vi "DAQ setting.vi"(8 "error in (no error)":errorcluster, 11 "vi reference":refnum<vi>) -> (0 "error Out":errorcluster, 3 "Out reference":refnum<vi>)   [LabVIEW 2015]
uses:
  Control Button/Exit.ctl
  Control Button/Save.ctl
  <vilib>/addons/database/Connection.llb/DB Tools Open Connec (String).vi
  <vilib>/addons/database/_DB Variant To Data/Database Variant To Data.xnode
  <vilib>/addons/database/NI_Database_API.lvlib
panel:
  out "error out":errorcluster
  in  "read":bool
  out "subarray":string[](array[string])
  in  "Save":T1
  in  "Exit":T2
  in  "Tab Control":T3(tab)
  in  "DAQmx OutPut Setting":T4
  in  "DAQmx InPut Setting":T5
  in  "DAQmx Analog Input Setting":T6
  in  "DAQmx  Counter In":tag
  in  "DAQmx  Counter In":tag
  in  "DAQmx Counter Out":tag
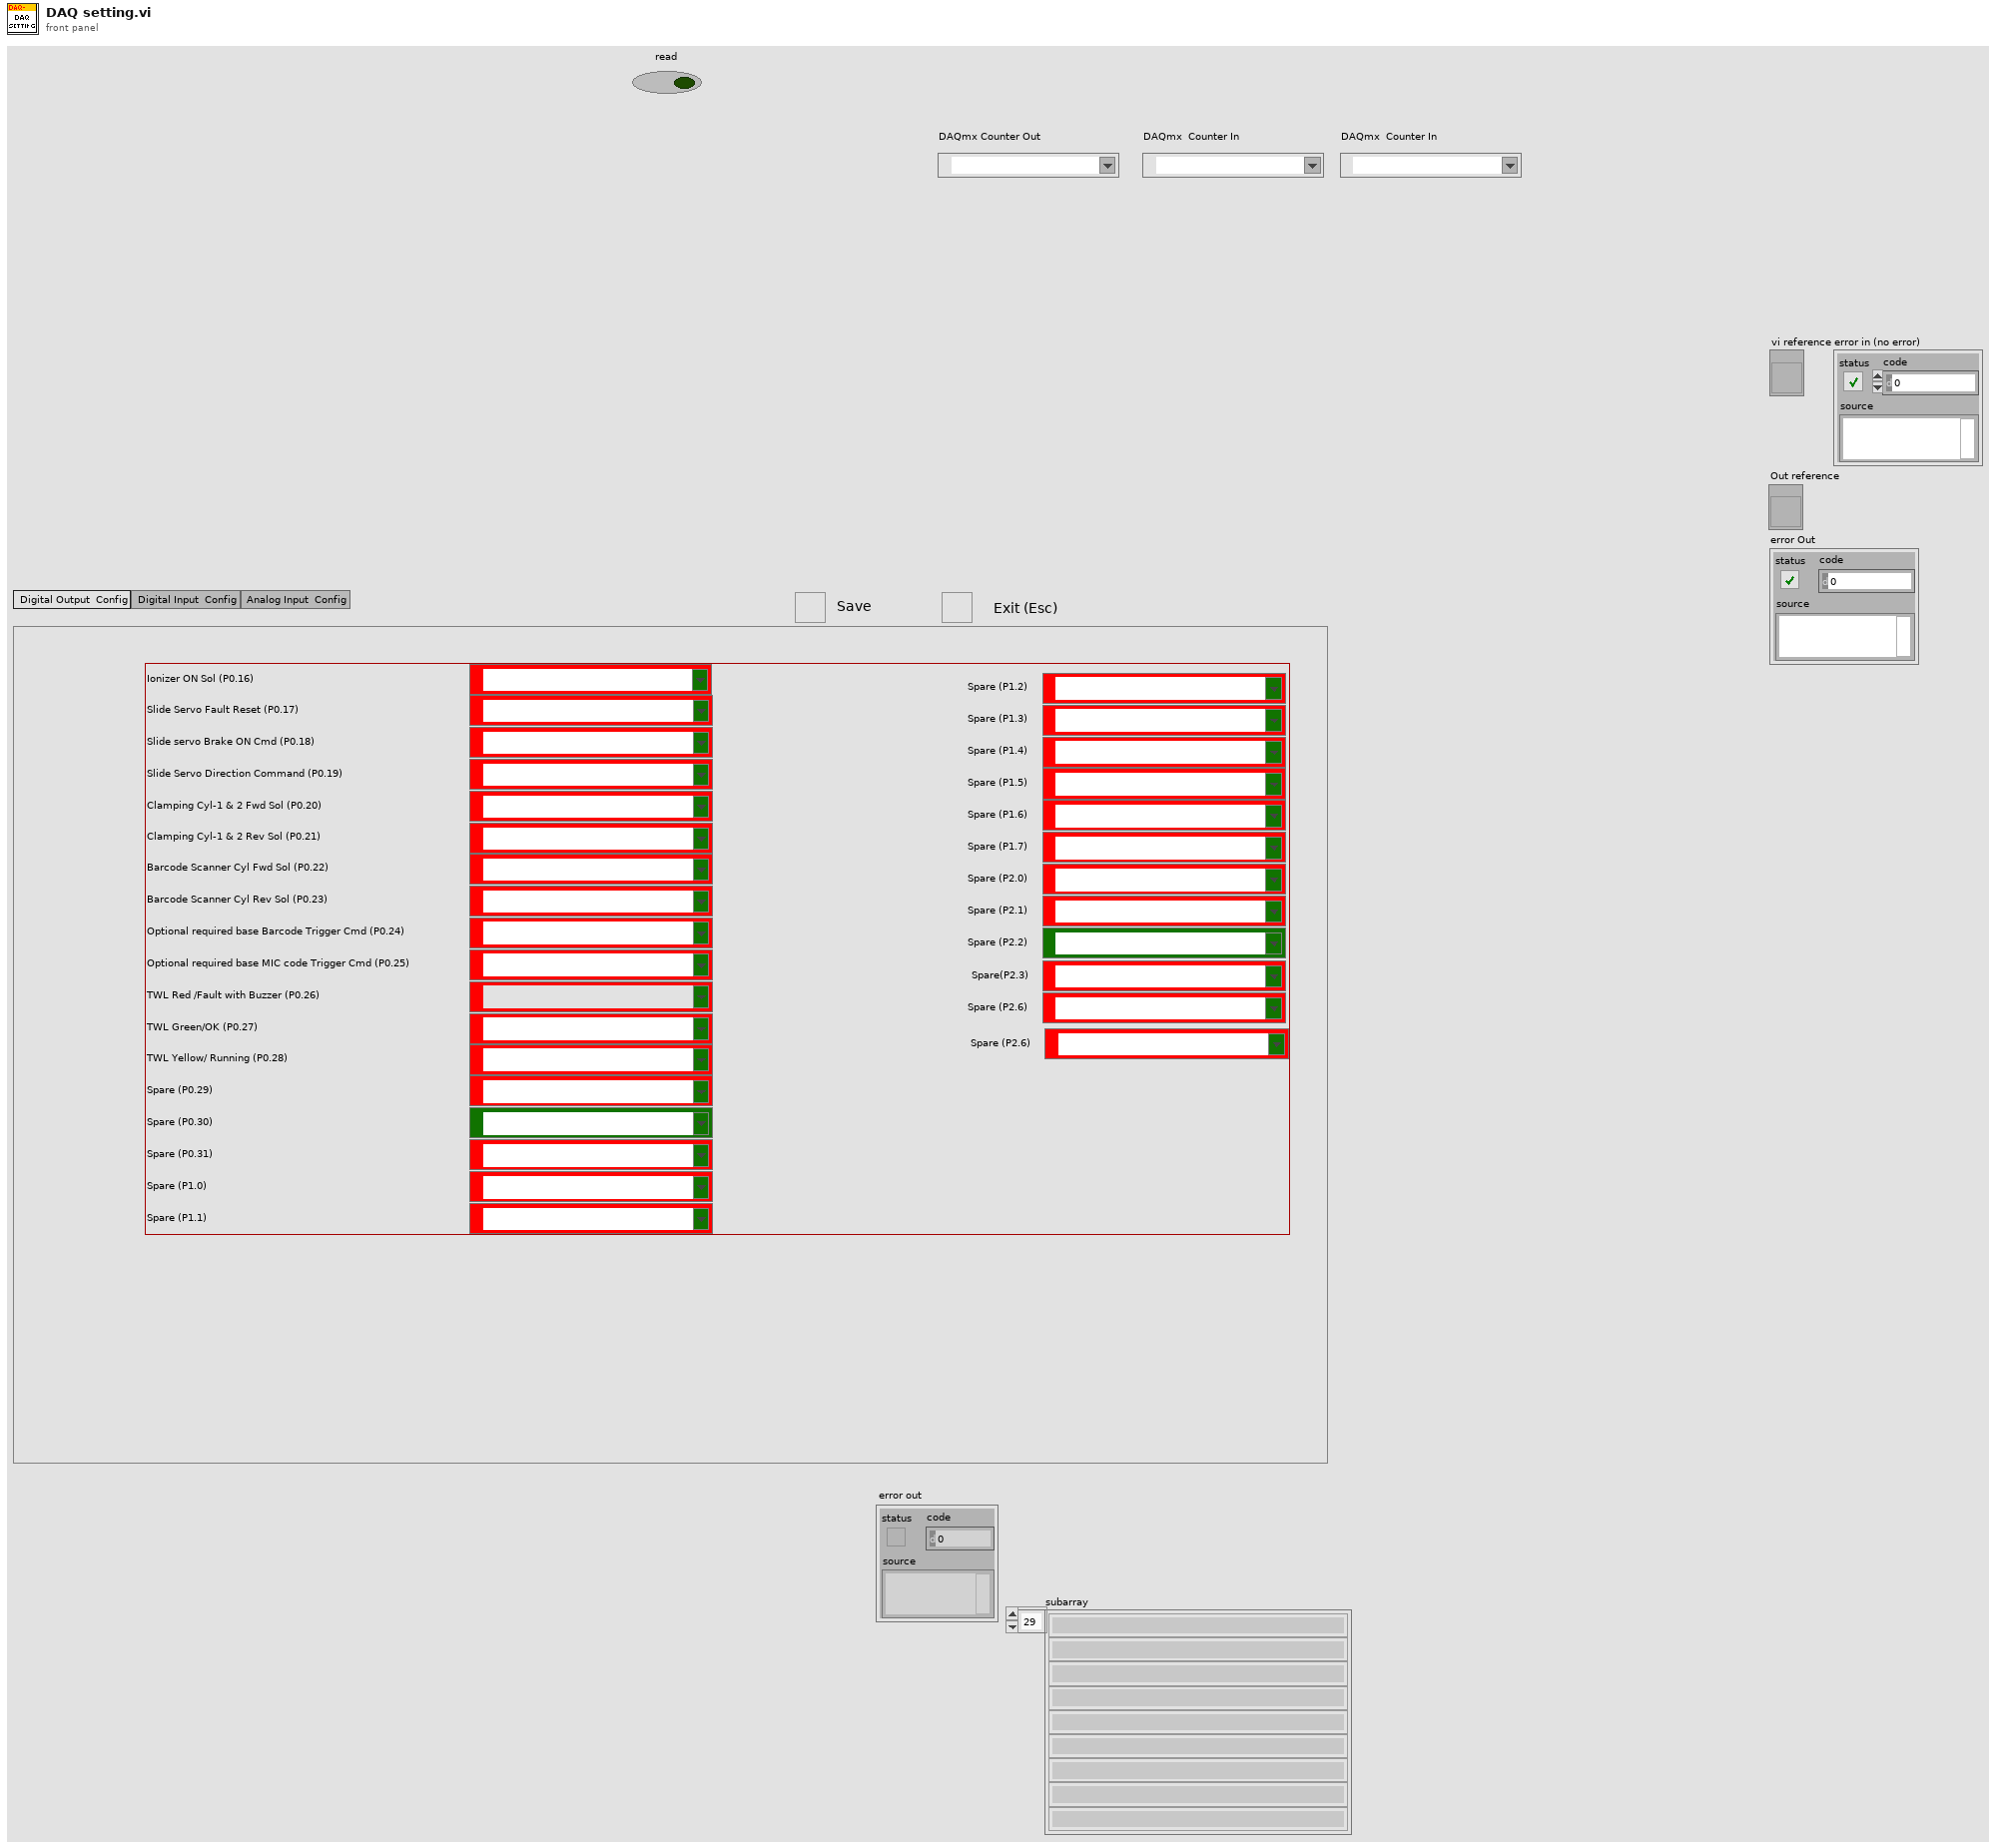
[diagram p1: front panel]
types:
  T1 = typedef "Save.ctl" = bool
  T2 = typedef "Exit.ctl" = bool
  T3 = enum32{"Digital Output  Config", "Digital Input  Config", "Analog Input  Config"}
  T4 = cluster{"DAQmx OutPut_00":tag, "DAQmx OutPut_01":tag, "DAQmx OutPut_02":tag, "DAQmx OutPut_03":tag, "DAQmx OutPut_04":tag, "DAQmx OutPut_05":tag, "DAQmx OutPut_06":tag, "DAQmx OutPut_07":tag, "DAQmx OutPut_08":tag, "DAQmx OutPut_09":tag, "DAQmx OutPut_10":tag, "DAQmx OutPut_11":tag, "DAQmx OutPut_12":tag, "DAQmx OutPut_13":tag, "DAQmx OutPut_14":tag, "DAQmx OutPut_15":tag, "DAQmx OutPut_16":tag, "DAQmx OutPut_17":tag, "DAQmx OutPut_18":tag, "DAQmx OutPut_19":tag, "DAQmx OutPut_20":tag, "DAQmx OutPut_21":tag, "DAQmx OutPut_22":tag, "DAQmx OutPut_23":tag, "DAQmx OutPut_12 2":tag, "DAQmx OutPut_13 2":tag, "DAQmx OutPut_14 2":tag, "DAQmx OutPut_15 2":tag, "DAQmx OutPut_16 2":tag, "String":string, "DAQmx OutPut_16 3":tag}
  T5 = cluster{"DAQmx InPut_00":tag, "DAQmx InPut_01":tag, "DAQmx InPut_02":tag, "DAQmx InPut_03":tag, "DAQmx InPut_04":tag, "DAQmx InPut_05":tag, "DAQmx InPut_06":tag, "DAQmx InPut_07":tag, "DAQmx InPut_08":tag, "DAQmx InPut_09":tag, "DAQmx InPut_10":tag, "DAQmx InPut_11":tag, "DAQmx InPut_12":tag, "DAQmx InPut_13":tag, "DAQmx InPut_14":tag, "DAQmx InPut_15":tag, "Key":string}
  T6 = cluster{"DAQmx Analog Input_00":tag, "DAQmx Analog Input_01":tag, "DAQmx Analog Input_02":tag, "DAQmx Analog Input_03":tag, "DAQmx Analog Input_04":tag, "DAQmx Analog Input_05":tag, "DAQmx Analog Input_06":tag, "DAQmx Analog Input_07":tag, "DAQmx Analog Input_08":tag, "DAQmx Analog Input_09":tag, "DAQmx Analog Input_10":tag, "DAQmx Analog Input_11":tag, "DAQmx Analog Input_12":tag, "DAQmx Analog Input_13":tag, "DAQmx Analog Input_14":tag, "DAQmx Analog Input_15":tag, "DAQmx Analog Input_16":tag, "DAQmx Analog Input_17":tag, "DAQmx Analog Input_18":tag, "DAQmx Analog Input_19":tag, "DAQmx Analog Input_20":tag, "DAQmx Analog Input_21":tag, "DAQmx Analog Input_22":tag, "DAQmx Analog Input_23":tag, "DAQmx Analog Input_24":tag, "DAQmx Analog Input_25":tag, "DAQmx Analog Input_26":tag, "DAQmx Analog Input_27":tag, "DAQmx Analog Input_28":tag, "DAQmx Analog Input_29":tag, "DAQmx Analog Input_30":tag, "DAQmx Analog Input_31":tag, "String 2":string}
  T7 = enum8{"Enabled", "Disabled", "Disabled and Grayed Out"}
  T8 = typedef "NI_Database_API.lvlib/Conn ObjectReference.ctl" = refnum<k1>
  T9 = cluster{"data[0]":string, "data[1]":string, "data[2]":string, "data[3]":string, "data[4]":string, "data[5]":string, "data[6]":string, "data[7]":string, "data[8]":string, "data[9]":string, "data[10]":string, "data[11]":string, "data[12]":string, "data[13]":string, "data[14]":string, "data[15]":string, "data[16]":string}
  T10 = cluster{"data[0]":string, "data[1]":string, "data[2]":string, "data[3]":string, "data[4]":string, "data[5]":string, "data[6]":string, "data[7]":string, "data[8]":string, "data[9]":string, "data[10]":string, "data[11]":string, "data[12]":string, "data[13]":string, "data[14]":string, "data[15]":string, "data[16]":string, "data[17]":string, "data[18]":string, "data[19]":string, "data[20]":string, "data[21]":string, "data[22]":string, "data[23]":string, "data[24]":string, "data[25]":string, "data[26]":string, "data[27]":string, "data[28]":string, "data[29]":string, "data[30]":string}
  T11 = cluster{"data[0]":string, "data[1]":string, "data[2]":string, "data[3]":string, "data[4]":string, "data[5]":string, "data[6]":string, "data[7]":string, "data[8]":string, "data[9]":string, "data[10]":string, "data[11]":string, "data[12]":string, "data[13]":string, "data[14]":string, "data[15]":string, "data[16]":string, "data[17]":string, "data[18]":string, "data[19]":string, "data[20]":string, "data[21]":string, "data[22]":string, "data[23]":string, "data[24]":string, "data[25]":string, "data[26]":string, "data[27]":string, "data[28]":string, "data[29]":string, "data[30]":string, "data[31]":string, "data[32]":string}
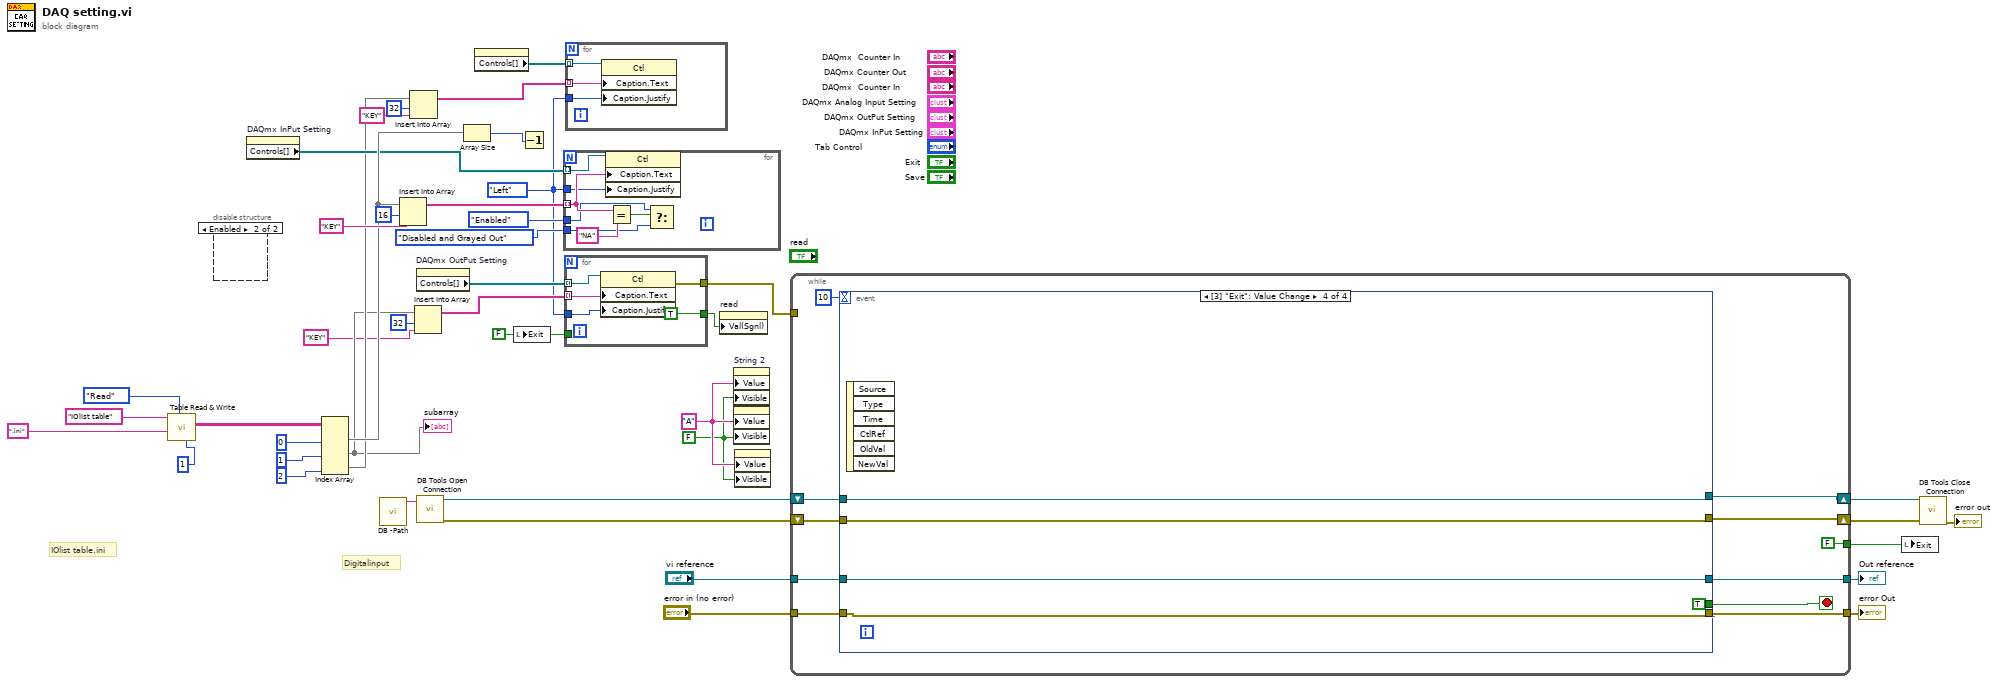
[diagram p0: block diagram]
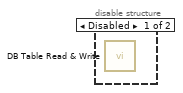
[diagram p2: hidden frame]
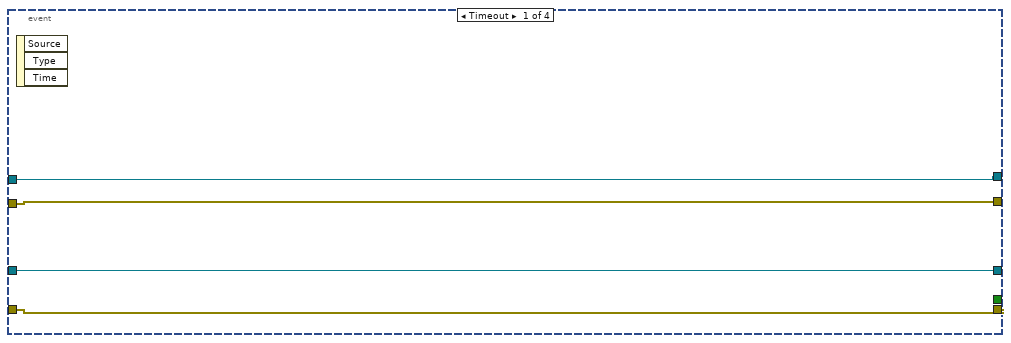
[diagram p3: hidden frame]
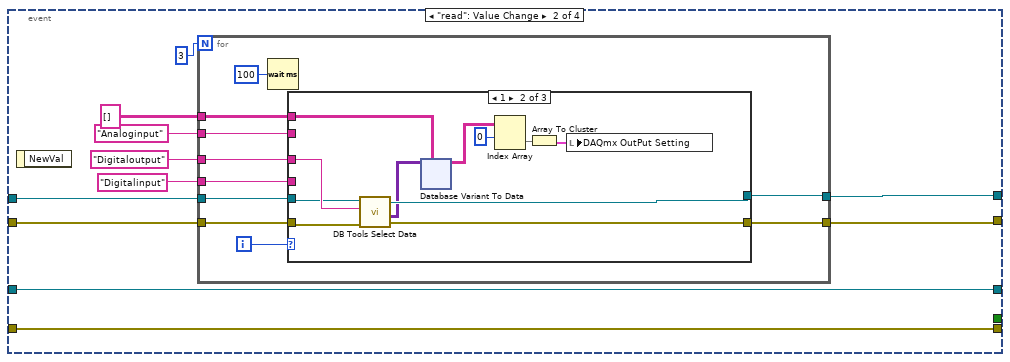
[diagram p4: hidden frame]
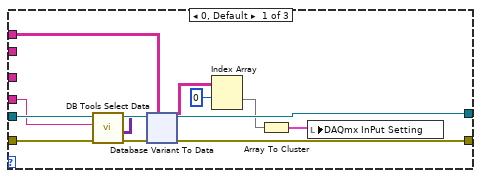
[diagram p5: hidden frame]
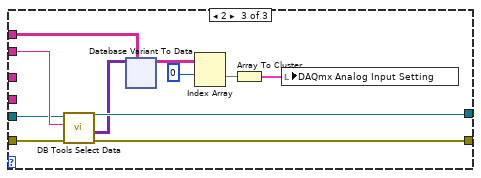
[diagram p6: hidden frame]
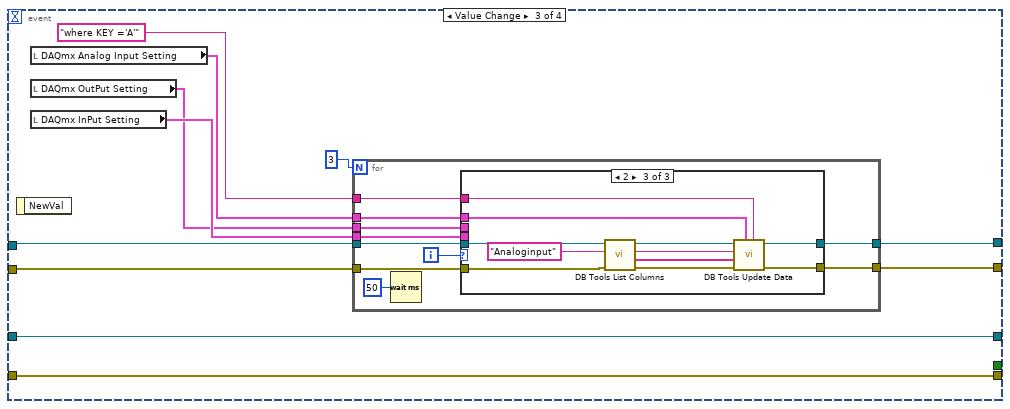
[diagram p7: hidden frame]
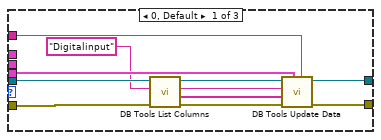
[diagram p8: hidden frame]
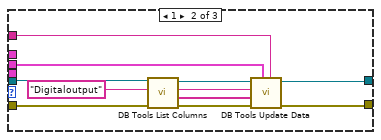
[diagram p9: hidden frame]
diagram:
  w1 = enum16{"Left", "Center", "Right"}."Left" ("Caption.Justification")
  w2 = FALSE ("Visible")
  w3 = "A" ("Value")
  w34 = T2 FALSE ("Exit")
  # "IOlist table.ini"
  # "Digitalinput"
  n1 = call "Table Read & Write.vi"("File Name"="IOlist table", "File type"=".ini", "Enum"=enum16{"Read", "Write"}."Read", "index"=1) -> ("Read Table"=w30:string[][])  [unwired: 5 in, 1 out]
  n2 = disable-structure shown="Enabled" {
    frame Disabled {
      n3 = call "DB Table Read & Write.vi"() -> ()  [unwired: 10 in, 2 out]
    }
    frame Enabled {
    }
  }
  n4 = property on="DAQmx InPut Setting" class="Clust (strict)"() -> ("Controls[]"=w13:refnum<vi>[])  [unwired: 2 in, 2 out]
  n5 = Index Array(array=w30, index (col) #1=0 ("disabled index (col)"), index (col) #2=1 ("index (col)"), index (col) #3=2 ("index (col)")) -> (element #1=w15:string[], element #2=w9:string[], element #3=w11:string[])  [unwired: 3 in]
  "subarray" <- w9
  n6 = call "DB -Path.vi"() -> ("String"=w27:string)  [unwired: 11 in]
  n7 = Insert Into Array(array=w15, index=16, new element="KEY" ("new element/subarray")) -> (w14:string[])
  n8 = Insert Into Array(array=w11, index=32, new element="KEY" ("new element/subarray")) -> (w4:string[])
  n9 = Insert Into Array(array=w9, index=32, new element="KEY" ("new element/subarray")) -> (w6:string[])
  n10 = property on="DAQmx OutPut Setting" class="Clust (strict)"() -> ("Controls[]"=w40:refnum<vi>[])  [unwired: 2 in, 2 out]
  n11 = call-poly <vilib>:"DB Tools Open Connection.vi"("connection information"=w27) -> ("error out"=w25:errorcluster, "connection reference"=w26:T8)  [unwired: 7 in]
  n12 = Array Size(array=w15) -> (size(s)=w18:i32)
  n13 = property on="DAQmx Analog Input Setting" class="Clust (strict)"() -> ("Controls[]"=w5:refnum<vi>[])  [unwired: 2 in, 2 out]
  n14 = local write "Exit"(w34) -> ()
  n15 = Decrement(x=w18) -> ()  [unwired: 1 out]
  n16 = for {
    tunnel: w13 -> [w50] mode=indexing
    tunnel: w14 -> [w48] mode=indexing
    tunnel: T7."Enabled" ("Disabled") -> [w47]
    tunnel: T7."Disabled and Grayed Out" ("Disabled") -> [w46]
    tunnel: w1 -> [w44]
    n17 = property class="Ctl"(reference=w50, "Caption.Text"=w48, "Caption.Justify"=w44) -> ()  [unwired: 1 in, 2 out]
    n18 = Equal?(x=w48, y="NA") -> (x = y?=w45:bool)
    n19 = Select(t=w47, s=w45, f=w46) -> ()  [unwired: 1 out]
  }
  n20 = for {
    tunnel: w40 -> [w55] mode=indexing
    tunnel: w6 -> [w54] mode=indexing
    tunnel: w34 -> [_]
    tunnel: [w53] -> w29
    tunnel: [TRUE] -> w28
    tunnel: w1 -> [w51]
    n21 = property class="Ctl"(reference=w55, "Caption.Text"=w54, "Caption.Justify"=w51) -> (error out=w53:errorcluster)  [unwired: 1 in, 1 out]
  }
  n22 = for {
    tunnel: w5 -> [w58] mode=indexing
    tunnel: w4 -> [w57] mode=indexing
    tunnel: w1 -> [w56]
    n23 = property class="Ctl"(reference=w58, "Caption.Text"=w57, "Caption.Justify"=w56) -> ()  [unwired: 1 in, 2 out]
  }
  n24 = property on="read" class="Bool (strict)"("Val(Sgnl)"=w28) -> ()  [unwired: 2 in, 2 out]
  n25 = property on="String 2" class="Str"("Value"=w3, "Visible"=w2) -> ()  [unwired: 2 in, 2 out]
  n26 = property on="Key" class="Str"("Value"=w3, "Visible"=w2) -> ()  [unwired: 2 in, 2 out]
  n27 = property on="String" class="Str"("Value"=w3, "Visible"=w2) -> ()  [unwired: 2 in, 2 out]
  n28 = while {
    tunnel: [FALSE] -> w39
    tunnel: "vi reference" -> [w66]
    tunnel: "error in (no error)" -> [w65]
    tunnel: [w64] -> w36
    tunnel: [w63] -> w35
    tunnel: w29 -> [_]
    shift-right: [w60] -> w24
    shift-left: w26 -> [w62]
    shift-right: [w59] -> w23
    shift-left: w25 -> [w61]
    stop <- w68 stop-if-true
    n29 = event shown="[3] \"Exit\": Value Change" {
      selector: _ -> [_ _ _ _]
      dyn-events: _ -> [_ _ _ _]
      timeout: 10 -> [_ _ _ _]
      tunnel: [_ _ _ TRUE] -> w68
      tunnel: w66 -> [w73 w84 w271 w315]
      tunnel: w65 -> [w72 w83 w270 w314]
      tunnel: [w73 w84 w271 w315] -> w64
      tunnel: [w72 w83 w270 w314] -> w63
      tunnel: w62 -> [w71 w77 w269 w313]
      tunnel: w61 -> [w70 w76 w268 w312]
      tunnel: [w71 w79 w266 w313] -> w60
      tunnel: [w70 w78 w265 w312] -> w59
      event Timeout {
        n30 = event-data() -> ()  [unwired: 1 in, 3 out]
      }
      event "read": Value Change {
        n31 = event-data() -> ()  [unwired: 1 in, 1 out]
        n32 = for {
          N: 3 -> [_]
          tunnel: "Digitalinput" ("table") -> [w92]
          tunnel: w77 -> [w91]
          tunnel: w76 -> [w90]
          tunnel: [w89] -> w79
          tunnel: [w88] -> w78
          tunnel: "Digitaloutput" ("table") -> [w87]
          tunnel: "Analoginput" ("table") -> [w86]
          tunnel: string[][] [] -> [w85]
          i -> [w94]
          n33 = Wait (ms)(milliseconds to wait=u32 100) -> ()  [unwired: 1 out]
          n34 = case shown="1" w94 {
            tunnel: w92 -> [w100 _ _]
            tunnel: w91 -> [w105 w160 w213]
            tunnel: w90 -> [w104 w159 w212]
            tunnel: [w103 w157 w211] -> w89
            tunnel: [w102 w156 w210] -> w88
            tunnel: w87 -> [_ w161 _]
            tunnel: w86 -> [_ _ w215]
            tunnel: w85 -> [w101 w158 w214]
            frame 0, Default {
              n35 = call <vilib>:"DB Tools Select Data.vi"("error in (no error)"=w104, "table"=w100, "connection reference"=w105) -> ("error out"=w95:errorcluster, "data"=w99:variant[][], "connection reference out"=w103:T8)  [unwired: 3 in]
              n36 = xnode "Database Variant To Data"("database variant"=w99, "error in (no error)"=w95, "type"=w101) -> ("data"=w98:string[][], "error out"=w102:errorcluster)
              n37 = Index Array(array=w98, index (row)=0) -> (element=w97:string[])  [unwired: 1 in]
              n38 = Array To Cluster(array=w97) -> (cluster=w96:T9)
              n39 = local write "DAQmx InPut Setting"(w96) -> ()
            }
            frame 1 {
              n40 = call <vilib>:"DB Tools Select Data.vi"("error in (no error)"=w159, "table"=w161, "connection reference"=w160) -> ("error out"=w156:errorcluster, "data"=w155:variant[][], "connection reference out"=w157:T8)  [unwired: 3 in]
              n41 = xnode "Database Variant To Data"("database variant"=w155, "type"=w158) -> ("data"=w154:string[][])  [unwired: 1 in, 1 out]
              n42 = Index Array(array=w154, index (row)=0 ("disabled index (col)")) -> (element=w152:string[])  [unwired: 1 in]
              n43 = Array To Cluster(array=w152) -> (cluster=w151:T10)
              n44 = local write "DAQmx OutPut Setting"(w151) -> ()
            }
            frame 2 {
              n45 = call <vilib>:"DB Tools Select Data.vi"("error in (no error)"=w212, "table"=w215, "connection reference"=w213) -> ("error out"=w210:errorcluster, "data"=w208:variant[][], "connection reference out"=w211:T8)  [unwired: 3 in]
              n46 = xnode "Database Variant To Data"("database variant"=w208, "type"=w214) -> ("data"=w209:string[][])  [unwired: 1 in, 1 out]
              n47 = Index Array(array=w209, index (row)=0 ("disabled index (col)")) -> (element=w207:string[])  [unwired: 1 in]
              n48 = Array To Cluster(array=w207) -> (cluster=w206:T11)
              n49 = local write "DAQmx Analog Input Setting"(w206) -> ()
            }
          }
        }
      }
      event Value Change {
        n50 = event-data() -> ()  [unwired: 1 in, 1 out]
        n51 = local read "DAQmx Analog Input Setting"() -> (w262:T6)
        n52 = local read "DAQmx OutPut Setting"() -> (w261:T4)
        n53 = local read "DAQmx InPut Setting"() -> (w267:T5)
        n54 = for {
          N: 3 -> [_]
          tunnel: w269 -> [w280]
          tunnel: w268 -> [w279]
          tunnel: w262 -> [w278]
          tunnel: w261 -> [w277]
          tunnel: w267 -> [w276]
          tunnel: [w275] -> w266
          tunnel: [w274] -> w265
          tunnel: "where KEY ='A'" -> [w272]
          i -> [w281]
          n55 = Wait (ms)(milliseconds to wait=u32 50) -> ()  [unwired: 1 out]
          n56 = case shown="2" w281 {
            tunnel: w280 -> [w288 w297 w311]
            tunnel: w279 -> [w287 w298 w306]
            tunnel: w278 -> [_ _ w308]
            tunnel: w277 -> [_ w299 _]
            tunnel: w276 -> [w289 _ _]
            tunnel: [w291 w301 w310] -> w275
            tunnel: [w290 w300 w309] -> w274
            tunnel: w272 -> [w282 w292 w302]
            frame 0, Default {
              w283 = "Digitalinput" ("table")
              n57 = call <vilib>:"DB Tools List Columns.vi"("error in (no error)"=w287, "table"=w283, "connection reference"=w288) -> ("error out"=w284:errorcluster, "columns"=w286:string[], "connection reference out"=w285:T8)  [unwired: 1 in, 1 out]
              n58 = call <vilib>:"DB Tools Update Data.vi"("condition"=w282, "data"=w289, "error in (no error)"=w284, "columns"=w286, "table"=w283, "connection reference"=w285) -> ("error out"=w290:errorcluster, "connection reference out"=w291:T8)  [unwired: 4 in]
            }
            frame 1 {
              w293 = "Digitaloutput" ("table")
              n59 = call <vilib>:"DB Tools List Columns.vi"("error in (no error)"=w298, "table"=w293, "connection reference"=w297) -> ("error out"=w296:errorcluster, "columns"=w294:string[], "connection reference out"=w295:T8)  [unwired: 1 in, 1 out]
              n60 = call <vilib>:"DB Tools Update Data.vi"("condition"=w292, "data"=w299, "error in (no error)"=w296, "columns"=w294, "table"=w293, "connection reference"=w295) -> ("error out"=w300:errorcluster, "connection reference out"=w301:T8)  [unwired: 4 in]
            }
            frame 2 {
              w304 = "Analoginput" ("table")
              n61 = call <vilib>:"DB Tools List Columns.vi"("error in (no error)"=w306, "table"=w304, "connection reference"=w311) -> ("error out"=w305:errorcluster, "columns"=w303:string[], "connection reference out"=w307:T8)  [unwired: 1 in, 1 out]
              n62 = call <vilib>:"DB Tools Update Data.vi"("condition"=w302, "data"=w308, "error in (no error)"=w305, "columns"=w303, "table"=w304, "connection reference"=w307) -> ("error out"=w309:errorcluster, "connection reference out"=w310:T8)  [unwired: 4 in]
            }
          }
        }
      }
      event Value Change {
        n63 = event-data() -> ()  [unwired: 1 in, 6 out]
      }
    }
  }
  "Out reference" <- w36
  "error Out" <- w35
  n64 = local write "Exit"(w39) -> ()
  n65 = call <vilib>:"DB Tools Close Connection.vi"("error in (no error)"=w23, "connection reference"=w24) -> ("error out"=→"error out":errorcluster)  [unwired: 5 in]
